vi "Data_Logger_System.vi"() -> ()   [LabVIEW 2020]
panel:
  in  "VISA resource name":refnum<visa-resource-name>
  in  "Table Control":string[][](table)
  out "Humidity":dbl(graph)
  out "Temperature":dbl(graph)
  out "Humidity":dbl(knob) scale=0.0..100.0
  out "Thermometer":dbl(slide) scale=0.0..100.0
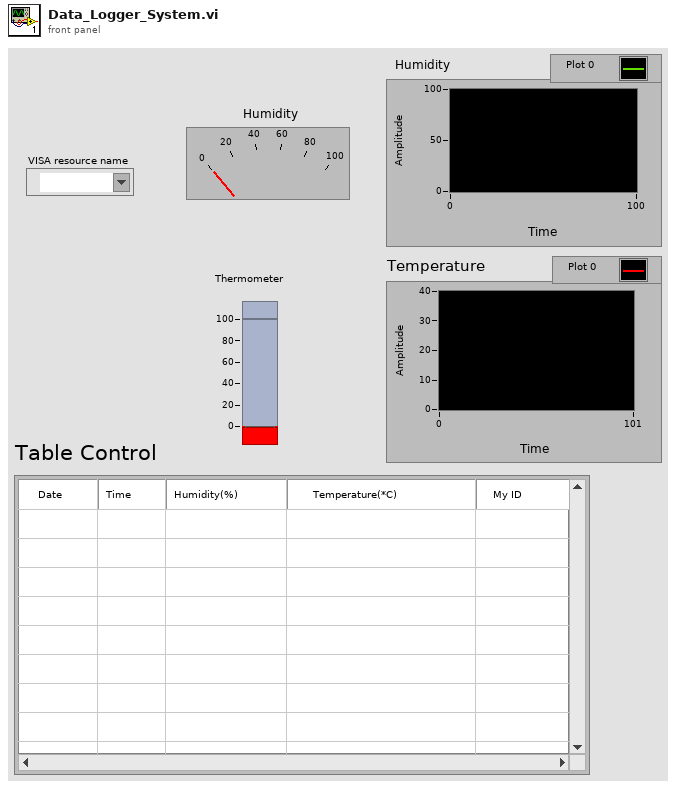
[diagram p1: front panel]
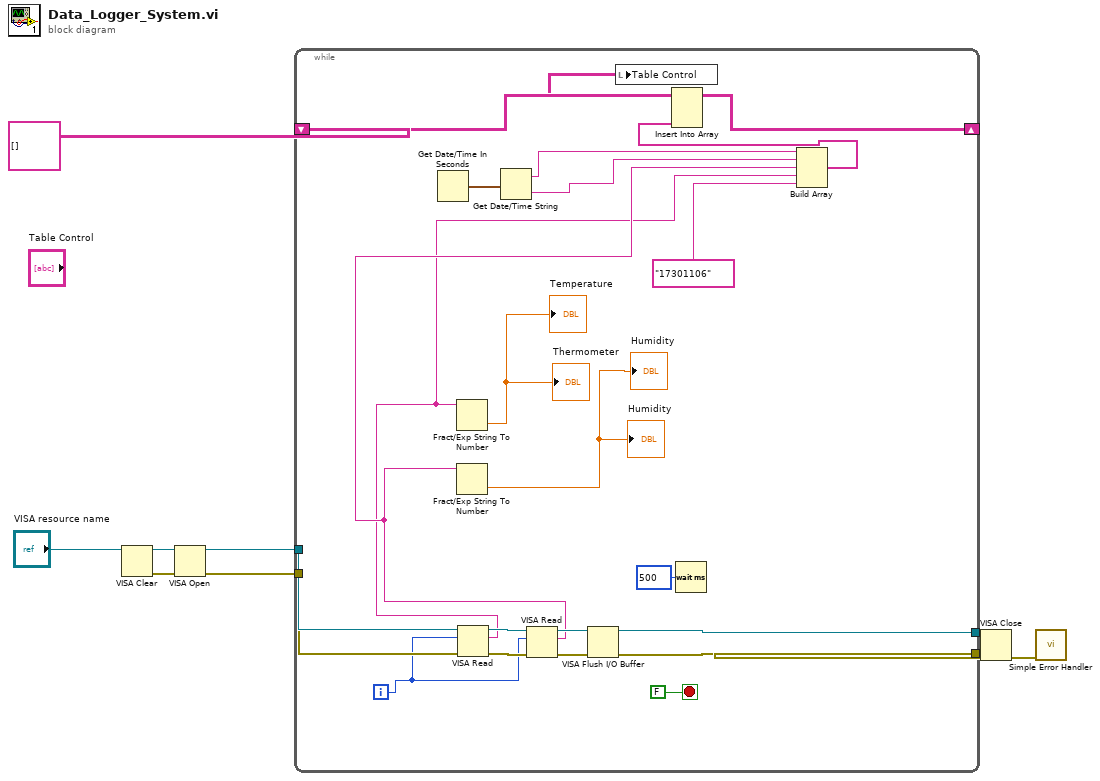
[diagram p0: block diagram]
diagram:
  n1 = VISA Clear(VISA resource name="VISA resource name") -> (VISA resource name out=w8:refnum<visa-resource-name>, error out=w9:errorcluster)  [unwired: 1 in]
  n2 = VISA Open(error in (no error)=w9, VISA resource name=w8) -> (VISA resource name=w6:refnum<visa-resource-name>, error out=w5:errorcluster)  [unwired: 3 in]
  n3 = while {
    tunnel: w6 -> [w31]
    tunnel: w5 -> [w30]
    tunnel: [w25] -> w4
    tunnel: [w24] -> w3
    shift-right: [w21] -> _
    shift-left: string[][] [] -> [w22]
    i -> [w23]
    stop <- FALSE stop-if-true
    n4 = Get Date/Time In Seconds() -> (seconds since 1Jan1904=w18:timestamp)
    n5 = VISA Read(VISA resource name=w31, byte count=w23, error in (no error)=w30) -> (VISA resource name out=w29:refnum<visa-resource-name>, read buffer=w10:string, error out=w28:errorcluster)  [unwired: 1 out]
    n6 = Fract/Exp String To Number(string=w10) -> (number=→"Thermometer" →"Temperature":dbl)  [unwired: 3 in, 1 out]
    n7 = Get Date/Time String(seconds (now)=w18) -> (date string=w17:string, time string=w16:string)  [unwired: 2 in]
    n8 = VISA Read(VISA resource name=w29, byte count=w23, error in (no error)=w28) -> (VISA resource name out=w26:refnum<visa-resource-name>, read buffer=w11:string, error out=w27:errorcluster)  [unwired: 1 out]
    n9 = Fract/Exp String To Number(string=w11) -> (number=→"Humidity" →"Humidity":dbl)  [unwired: 3 in, 1 out]
    n10 = VISA Flush I/O Buffer(VISA resource name=w26, error in (no error)=w27) -> (VISA resource name out=w25:refnum<visa-resource-name>, error out=w24:errorcluster)  [unwired: 1 in]
    n11 = Wait (ms)(milliseconds to wait=u32 500) -> ()  [unwired: 1 out]
    n12 = Build Array(w17, w16, w11, w10, "17301106" ("element")) -> (w12:string[])
    n13 = Insert Into Array(array=w22, new element=w12) -> (w21:string[][])  [unwired: 2 in]
    n14 = local write "Table Control"(w21) -> ()
  }
  n15 = VISA Close(VISA resource name=w4, error in (no error)=w3) -> (error out=w7:errorcluster)
  n16 = call <vilib>:"Simple Error Handler.vi"("error in (no error)"=w7) -> ()  [unwired: 4 in, 5 out]
